vi "event_animal_ID.vi"(5 "NewVal":u16, 7 "OldVal":u16, 8 "error in":errorcluster, 9 "reference cluster in":T1, 11 "Digital in":refnum<vi>) -> (0 "error out":errorcluster)   [LabVIEW 2016]
uses:
  Type Definitions/reference_cluster.ctl
  Type Definitions/vars_settings.ctl
  Type Definitions/stim_type.ctl
  Type Definitions/backlight_type.ctl
  Type Definitions/vars_runtime.ctl
  Type Definitions/data.ctl
  Type Definitions/notifier_elements_GUI.ctl
  Type Definitions/notifier_elements_DAQ.ctl
  Type Definitions/notifier_elements_write.ctl
  Type Definitions/control_references.ctl
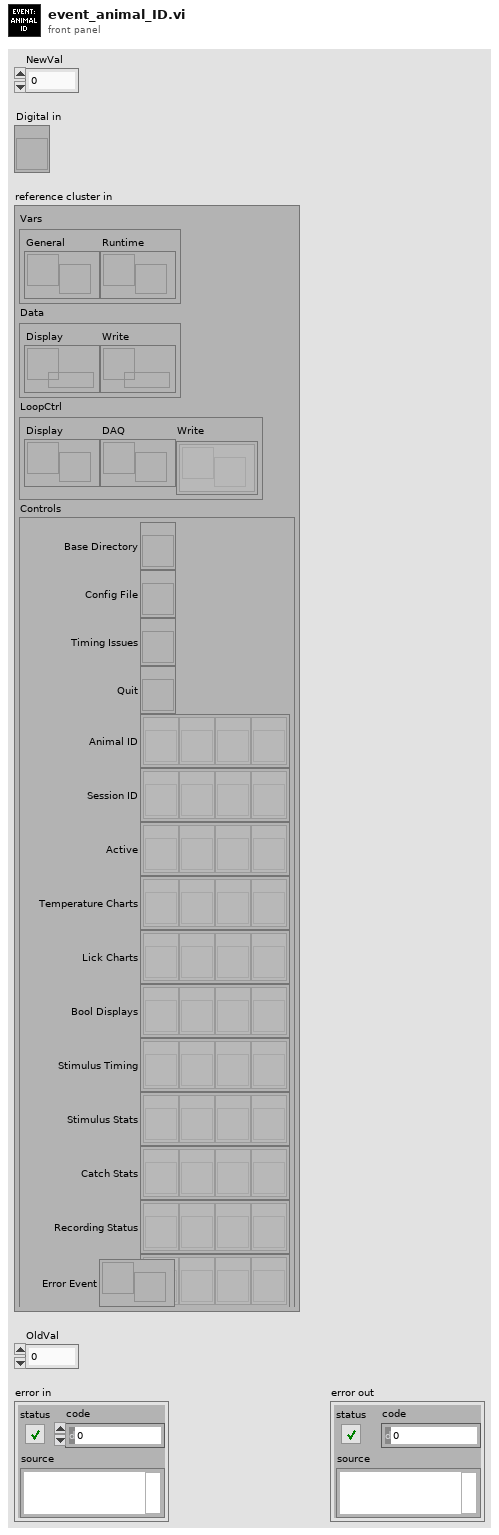
[diagram p1: front panel]
types:
  T1 = typedef "reference_cluster.ctl" = cluster{"Vars":cluster{"General":refnum<notifier>, "Runtime":refnum<notifier>}, "Data":cluster{"Display":refnum<queue>, "Write":refnum<queue>}, "LoopCtrl":cluster{"Display":refnum<notifier>, "DAQ":refnum<notifier>, "Write":refnum<notifier>[]}, "Controls":T2, "Error Event":refnum<user-event>}
  T2 = typedef "control_references.ctl" = cluster{"Base Directory":refnum<vi>, "Config File":refnum<vi>, "Timing Issues":refnum<vi>, "Quit":refnum<vi>, "Animal ID":refnum<vi>[], "Session ID":refnum<vi>[], "Active":refnum<vi>[], "Temperature Charts":refnum<vi>[], "Lick Charts":refnum<vi>[], "Bool Displays":refnum<vi>[], "Stimulus Timing":refnum<vi>[], "Stimulus Stats":refnum<vi>[], "Catch Stats":refnum<vi>[], "Recording Status":refnum<vi>[], "Pairing":refnum<vi>[]}
  T3 = typedef "vars_settings.ctl" = cluster{"base directory":path, "data directory":path, "active":bool, "running":bool, "pairing":bool, "clean tubes":bool, "animal ID":u16, "session ID":u16, "base temp":dbl, "d wait min":u16, "d wait max":u16, "d timeout":u16, "d timeout catch":u16, "d reward":u16, "n reward":u16, "idx stim":u16, "timeout win":u16, "lick win":i32[], "stim type":T4[], "stim dur":u16[], "stim amp":dbl[], "stim freq":u16[], "stim ramp":u16[], "stim catch":u8[], "pairing delay":i16[], "square dur":u16[], "square delay":i16[], "square freq":u8[], "square dc":u8[], "stim shape":dbl[][], "square shape":bool[][], "backlight type":T5, "backlight freq":u16, "dStimOne dur":u16[], "dStimOne delay":i16[], "dStimTwo dur":u16[], "dStimTwo delay":i16[]}
  T4 = typedef "stim_type.ctl" = enum16{"pulse", "vibration", "square", "sine"}
  T5 = typedef "backlight_type.ctl" = enum16{"none", "random", "regular"}
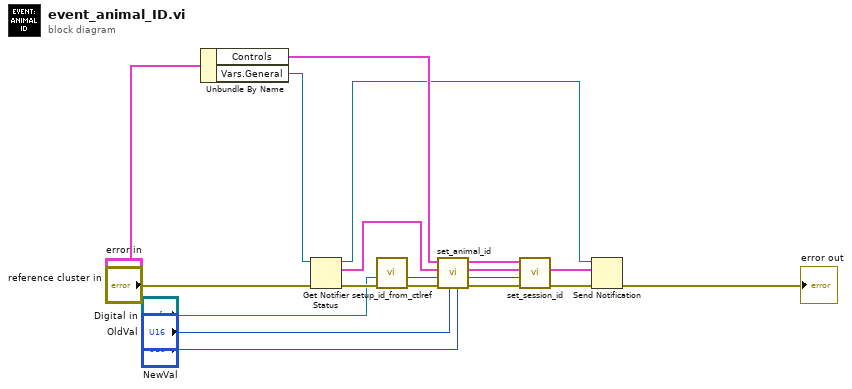
[diagram p0: block diagram]
diagram:
  n1 = Unbundle By Name("reference cluster in") -> ("Controls"=w16:T2, "Vars.General"=w6:refnum<notifier>)
  n2 = Get Notifier Status(notifier=w6, error in (no error)="error in") -> (notifier out=w9:refnum<notifier>, current notification=w13:T3[], error out=w8:errorcluster)  [unwired: 2 out]
  n3 = call "setup_id_from_ctlref.vi"("error in"=w8, "Ctl Refnum"="Digital in") -> ("error out"=w2:errorcluster, "setup ID"=w17:u16)  [unwired: 6 in]
  n4 = call "set_animal_id.vi"("new animal ID"="NewVal", "old animal ID"="OldVal", "error in"=w2, "setup ID"=w17, "settings array in"=w13, "control cluster in"=w16) -> ("error out"=w3:errorcluster, "setup ID"=w18:u16, "settings array out"=w14:T3[], "control cluster out"=w15:T2)
  n5 = call "set_session_id.vi"("control cluster in"=w15, "settings in"=w14, "setup ID"=w18, "error in"=w3) -> ("settings out"=w12:T3[], "error out"=w10:errorcluster)  [unwired: 3 in, 2 out]
  n6 = Send Notification(notification=w12, notifier=w9, error in (no error)=w10) -> (error out=→"error out":errorcluster)  [unwired: 1 out]
